vi "TestbenchWithCircuit.vi"() -> ()   [LabVIEW 2017]
uses:
  <vilib>/Simulation/Scripting/Companion Diagram/SimConfigNode/SimParams.ctl
  <vilib>/Simulation/Scripting/Companion Diagram/SimConfigNode/_simSolvers.ctl
  <vilib>/Simulation/Implementation/Shared/SIMSCR Execution Mode.ctl
  <vilib>/Simulation/Param Hierarchy/Typedefs/SIMPH Param Control Actions.ctl
  <vilib>/Simulation/Scripting/Editor Utilities/SIM subVI tag data.ctl
  <vilib>/Simulation/Scripting/Editor Utilities/SIM subVI execution type.ctl
  <vilib>/Simulation/Implementation/Shared/NILVSim_ParamChanged.vi
  <vilib>/Simulation/Implementation/Shared/NILVSIM_BeginStep.vi
  <vilib>/Simulation/Utility/Implementation/NILVSim Memory.llb/NILVSim Memory (core).vi
  <vilib>/Simulation/Implementation/Shared/SIM Fire Discrete SubVI.vi
  <vilib>/Simulation/Implementation/Shared/NILVSim_Manager.vi
  <vilib>/Utility/error.llb/Clear Errors.vi
  <vilib>/Simulation/Implementation/Shared/NILVSim_FinalizeModel.vi
  <vilib>/Simulation/Implementation/Shared/SIM Fire Discrete SubVI (Core).vi
  <vilib>/Simulation/Implementation/Shared/SIM Unbundle Sim Info.vi
  <vilib>/Simulation/Implementation/Shared/NILVSim_Initialize.vi
  <vilib>/rvi/DesktopExecutionNode/Execution/niFpgaDEN_Execute.vi
  <vilib>/Simulation/Utility/Implementation/NILVSim Get Time and IsAcceptedStep.vi
  <vilib>/Simulation/Implementation/Shared/SIMSH Read Queue.vi
  <vilib>/Simulation/Implementation/Shared/NILVSim_GetModelError.vi
  <vilib>/Simulation/Implementation/Shared/SIM Bundle Sim Info.vi
  <vilib>/Simulation/Scripting/Companion Diagram/SimConfigNode/SimDog.xnode
  <vilib>/Simulation/Implementation/XNodeFramework/SimXNode/SimX.xnode
  <vilib>/Simulation/EMI/Plugins/Multisim Design/MultisimEMICtrl.dll
  <vilib>/rvi/DesktopExecutionNode/DesktopExecutionNode.xnode
  <vilib>/Simulation/Implementation/Shared/NI_SIM_Implementation.lvlib
panel:
  in  "Tab Control":T1(tab)
  out "Iabc":dbl[][](graph)
  out "Vacb":dbl[][](graph)
  out "PLL to Grid":dbl[][](graph)
  out "Measured Frequency":dbl
  out "DC Link Info":dbl[][](graph)
  in  "enable":bool
  in  "reset":bool
  out "SwitchPositions":T2
  in  "setpoints":T3
  in  "parameters":T4={"PLL gain change"=FALSE, "PLL PI Kp"=25.0, "PLL PI Ki"=100.0, "wL factor"=0.01, "ExpectedFreq"=60.0, "AntiIslandingGain"=0.0, "VDCLink PI Kp"=-0.1, "VDCLink PI Ki*Ts"=-1e-07, "VDCLink PI output max"=1.0, "VDCLink PI output min"=-1.0, "ID PI Kp"=0.1, "ID PI Ki*Ts"=1e-07, "ID PI output max"=0.8, "ID PI output min"=-0.8, "IQ PID Kp"=0.1, "IQ PID Ki*Ts"=1e-07, "IQ PID output max"=0.5, "IQ PID output min"=-0.5, "ABC command scaling factor"=0.25}
  in  "SwitchConfig":T5={"DeadtimeTicks"=2, "triangle increment"=0.0014999997802078724}
  out "intermediate results":T6
  out "Waveform Chart":cluster{"A":sgl, "B":sgl, "C":sgl}(graph)
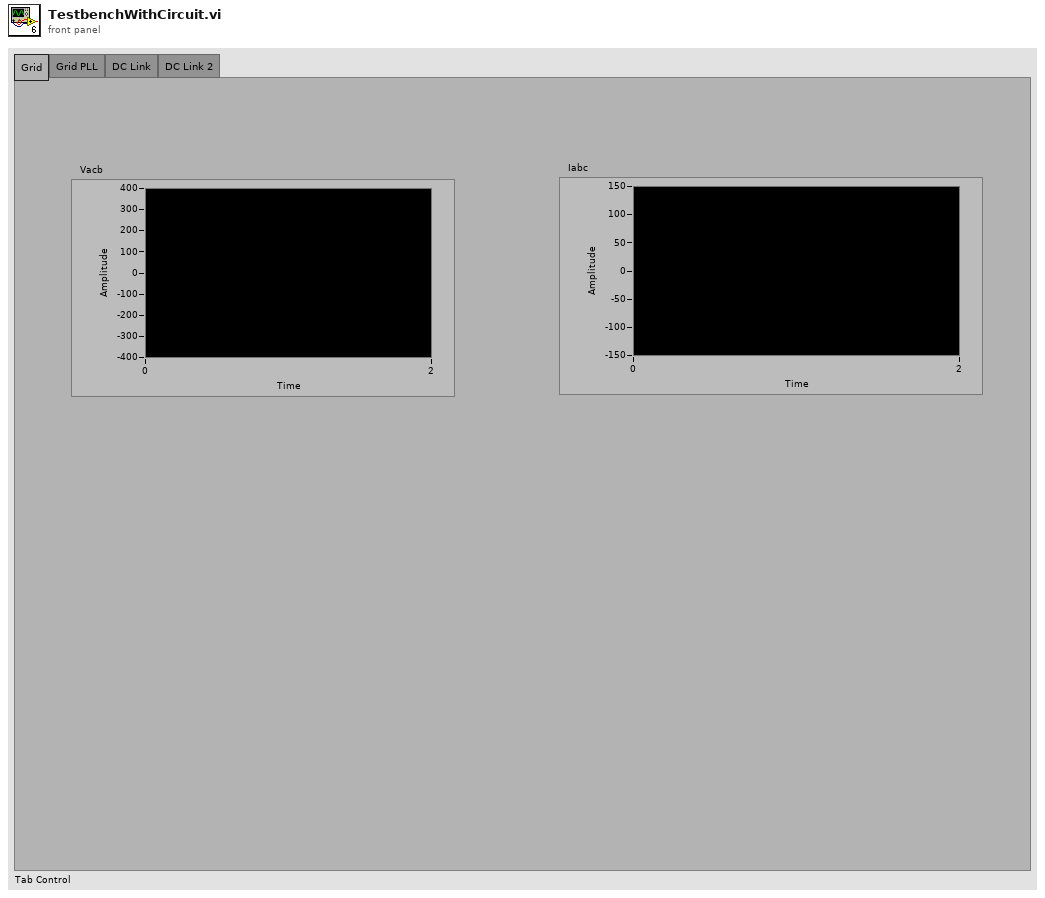
[diagram p1: front panel]
types:
  T1 = enum32{"Grid", "Grid PLL", "DC Link", "DC Link 2"}
  T2 = cluster{"UTop":bool, "UBottom":bool, "VTop":bool, "VBottom":bool, "WTop":bool, "WBottom":bool}
  T3 = cluster{"SetpntDCLink":sgl, "ID setpt":sgl, "override ID?":bool}
  T4 = cluster{"PLL gain change":bool, "PLL PI Kp":sgl, "PLL PI Ki":sgl, "wL factor":sgl, "ExpectedFreq":sgl, "AntiIslandingGain":sgl, "VDCLink PI Kp":sgl, "VDCLink PI Ki*Ts":sgl, "VDCLink PI output max":sgl, "VDCLink PI output min":sgl, "ID PI Kp":sgl, "ID PI Ki*Ts":sgl, "ID PI output max":sgl, "ID PI output min":sgl, "IQ PID Kp":sgl, "IQ PID Ki*Ts":sgl, "IQ PID output max":sgl, "IQ PID output min":sgl, "ABC command scaling factor":sgl}
  T5 = cluster{"DeadtimeTicks":u8, "triangle increment":fxp<+/-,32,1>}
  T6 = cluster{"V D Cmd":sgl, "V Q Cmd":sgl, "VGrid D":sgl, "VGrid Q":sgl, "IGrid D":sgl, "IGrid Q":sgl, "MeasuredFreq":sgl, "phase (pi)":sgl}
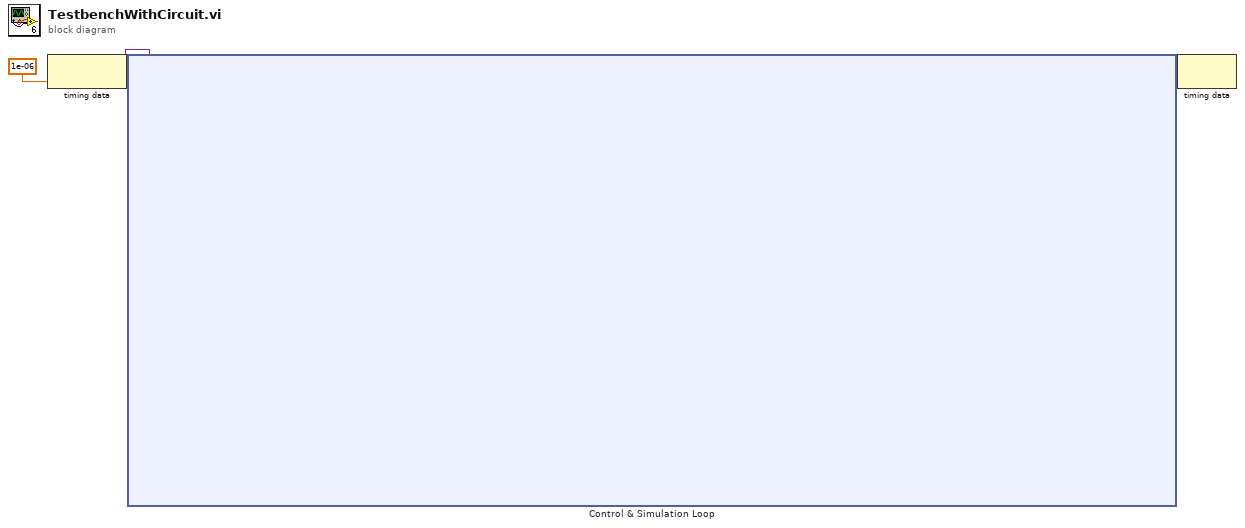
[diagram p0: block diagram]
diagram:
  n1 = node-c288(1e-06 ("Step Size (s)")) -> (w3:variant)
  n2 = node-c254 "Control & Simulation Loop"(w3) -> (w2:variant)
  n3 = node-c288(w2) -> ()  [unwired: 1 out]
